vi "Distance and Angle.vi"(8 "END":cluster{"X":dbl, "Y":dbl}, 11 "START":cluster{"X":dbl, "Y":dbl}) -> (2 "Angle":dbl, 3 "Distance":dbl)   [LabVIEW 2015]
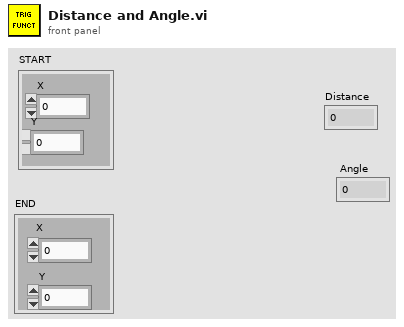
[diagram p1: front panel]
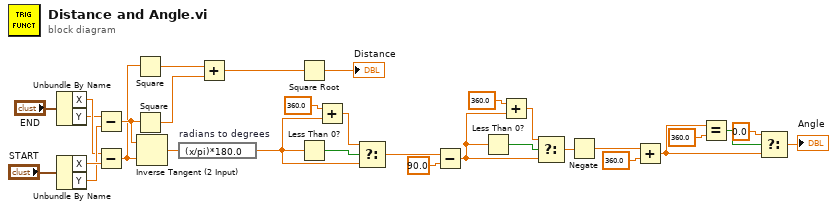
[diagram p0: block diagram]
diagram:
  n1 = Unbundle By Name("END") -> ("X"=w27:dbl, "Y"=w26:dbl)
  n2 = Unbundle By Name("START") -> ("X"=w29:dbl, "Y"=w28:dbl)
  n3 = Subtract(x=w26, y=w28) -> (x-y=w20:dbl)
  n4 = Subtract(x=w27, y=w29) -> (x-y=w19:dbl)
  n5 = Square(x=w19) -> (x^2=w25:dbl)
  n6 = Square(x=w20) -> (x^2=w24:dbl)
  n7 = Inverse Tangent (2 Input)(1:w19, 2:w20) -> (0:w21:dbl)
  n8 = expression code="(x/pi)*180.0" "radians to degrees"(w21) -> (w16:dbl)
  n9 = Add(x=w25, y=w24) -> (x+y=w23:dbl)
  n10 = Square Root(x=w23) -> (sqrt(x)=→"Distance":dbl)
  n11 = Less Than 0?(x=w16) -> (x < 0?=w18:bool)
  n12 = Add(x=360.0, y=w16) -> (x+y=w15:dbl)
  n13 = Select(t=w15, s=w18, f=w16) -> (s? t:f=w14:dbl)
  n14 = Subtract(x=w14, y=90.0) -> (x-y=w10:dbl)
  n15 = Less Than 0?(x=w10) -> (x < 0?=w12:bool)
  n16 = Add(x=360.0, y=w10) -> (x+y=w9:dbl)
  n17 = Select(t=w9, s=w12, f=w10) -> (s? t:f=w8:dbl)
  n18 = Negate(x=w8) -> (-x=w7:dbl)
  n19 = Add(x=w7, y=360.0) -> (x+y=w3:dbl)
  n20 = Equal?(x=w3, y=360.0) -> (x = y?=w4:bool)
  n21 = Select(t=0.0, s=w4, f=w3) -> (s? t:f=→"Angle":dbl)
